vi "MaxVelocityConstraint_getMaxVelocity.vi"(8 "Velocity":dbl, 9 "Curvature":dbl, 10 "statePose":T2={"TRANSLATION"={"X"=0.0, "Y"=0.0}, "ROTATION"={"VALUE"=0.0, "COS"=1.0, "SIN"=0.0}} {"ROTATION"."SIN" format="%13.4f"; "ROTATION"."COS" format="%13.4f"; "ROTATION"."VALUE" format="%13.4f"; "TRANSLATION"."Y" format="%14.3f"; "TRANSLATION"."X" format="%14.3f"}, 11 "MAX_VELOCITY_CONSTRAINT":T1 {"Max Velocity" format="%20.4f"}) -> (3 "absMaxVelocity":dbl)   [LabVIEW 2019, in "Trajectory_Library.lvlib"]
doc: "Return the maximum allowed velocity given the provided conditions.\n\nCalculation comments.\n // ac = v^2 / r\n // k (curvature) = 1 / r\n\n // therefore, ac = v^2 * k\n // ac / k = v^2\n // v = std::sqrt(ac / k)\n\n\nParameters:\n - CentripitalAccelConstraint - Constraint data structure\n - statePose - current traj state Pose\n - curvature - current traj curvature\n - maxVelocity - current traj max velocity\n\nReturns\n - maxVelocity - Maximum allowed velocity."
uses:
  Trajectory_Library.lvlib
  TypeDef/POSE2D.ctl
  TypeDef/TRANSLATION2D.ctl
  TypeDef/ROTATION2D.ctl
  TypeDef/TRAJ_CONSTRAINT_MAX_VELOCITY.ctl
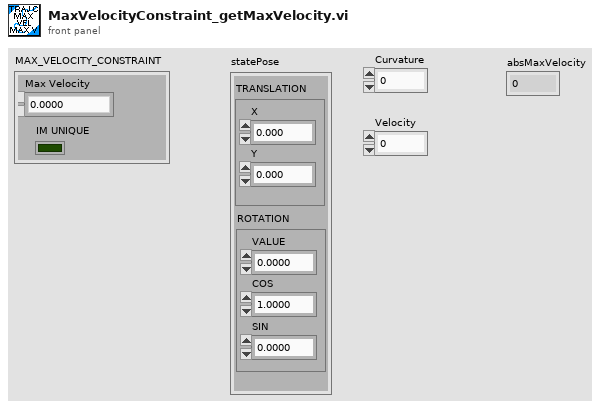
[diagram p1: front panel]
types:
  T1 = typedef "Trajectory_Library.lvlib/TRAJ_CONSTRAINT_MAX_VELOCITY.ctl" = cluster{"Max Velocity":dbl, "IM UNIQUE":bool}
  T2 = typedef "Trajectory_Library.lvlib/POSE2D.ctl" = cluster{"TRANSLATION":T3, "ROTATION":T4}
  T3 = typedef "Trajectory_Library.lvlib/TRANSLATION2D.ctl" = cluster{"X":dbl, "Y":dbl}
  T4 = typedef "Trajectory_Library.lvlib/ROTATION2D.ctl" = cluster{"VALUE":dbl, "COS":dbl, "SIN":dbl}
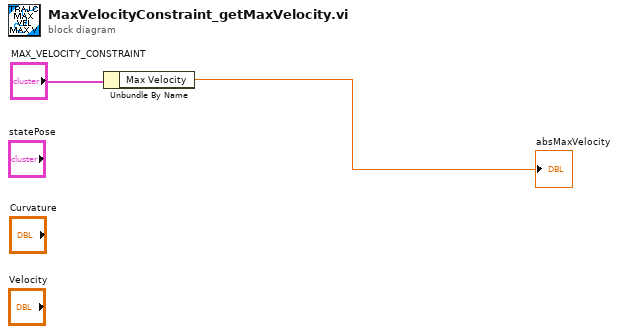
[diagram p0: block diagram]
diagram:
  n1 = Unbundle By Name("MAX_VELOCITY_CONSTRAINT") -> ("Max Velocity"=→"absMaxVelocity":dbl)
